vi "Write Setpoint.vi"(8 "error in (no error)":errorcluster, 10 "ILC in":refnum<class "ILC.lvclass">, 11 "ILC Actuator Cylinder in":refnum<class "ILC Actuator Cylinder.lvclass">) -> (0 "error out":errorcluster, 1 "Cylinder Results":T1, 2 "ILC out":refnum<class "ILC.lvclass">, 3 "ILC Actuator Cylinder out":refnum<class "ILC Actuator Cylinder.lvclass">)   [LabVIEW 2015, in "ILC Actuator Cylinder.lvclass"]
uses:
  ILC Actuator Cylinder.lvclass
  <userlib>/Common/ILC/ILC/ILC.lvclass
  Typedefs/Cylinder Results.ctl
  ILC Actuator Cylinder.lvclass/ILC Actuator Cylinder.ctl
  ILC DAC/ILC DAC/ILC DAC.lvclass
  Calculators/Force To Pressure Servo Valve Voltage/Force To Pressure Servo Valve Voltage.lvclass
  Typedefs/FAMT Typedefs.lvlib
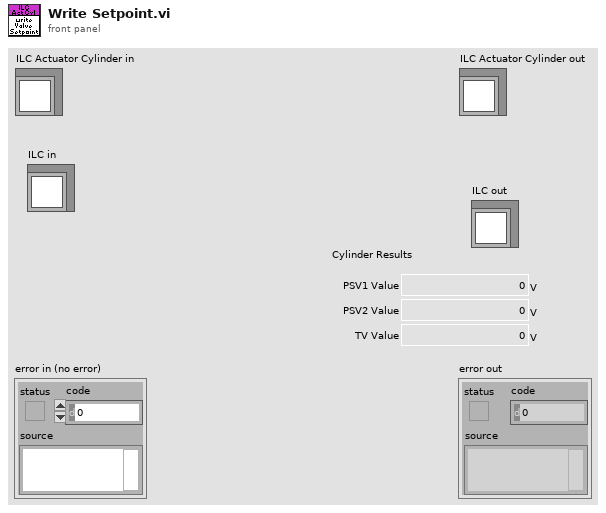
[diagram p1: front panel]
types:
  T1 = typedef "FAMT Typedefs.lvlib/Cylinder Results.ctl" = cluster{"PSV1 Value":dbl[unit], "PSV2 Value":dbl[unit], "TV Value":dbl[unit]}
  T2 = typedef "FAMT Typedefs.lvlib/Pressure Servo Valve Settings.ctl" = cluster{"Center Point":dbl[unit], "Area":dbl, "PA to PSI":dbl, "Off Value":dbl}
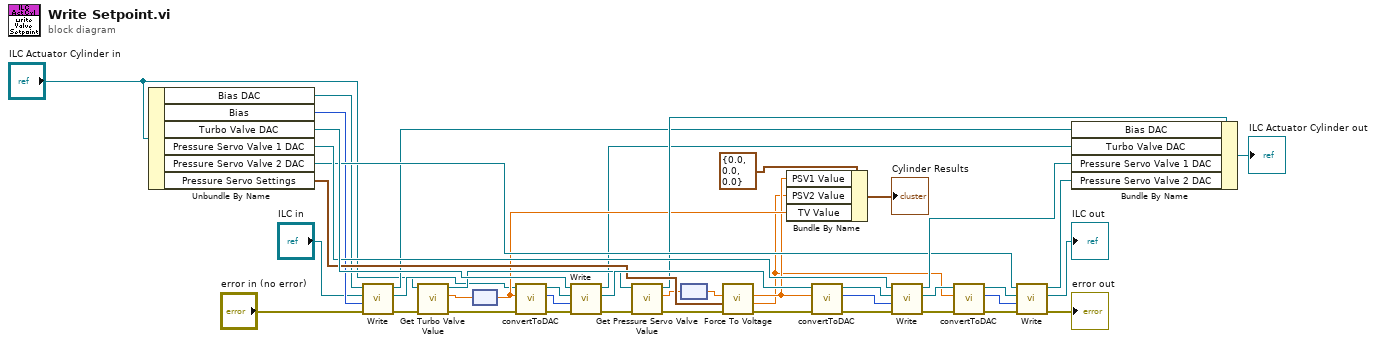
[diagram p0: block diagram]
diagram:
  n1 = Unbundle By Name("ILC Actuator Cylinder in") -> ("Bias DAC"=w9:refnum<class "ILC DAC.lvclass">, "Bias"=w6:u16, "Turbo Valve DAC"=w40:refnum<class "ILC DAC.lvclass">, "Pressure Servo Valve 1 DAC"=w37:refnum<class "ILC DAC.lvclass">, "Pressure Servo Valve 2 DAC"=w31:refnum<class "ILC DAC.lvclass">, "Pressure Servo Settings"=w24:T2)
  n2 = call-dynamic "Write.vi"("error in (no error)"="error in (no error)", "Value"=w6, "ILC in"="ILC in", "ILC DAC in"=w9) -> ("error out"=w2:errorcluster, "ILC out"=w4:refnum<class "ILC.lvclass">, "ILC DAC out"=w8:refnum<class "ILC DAC.lvclass">)  [unwired: 5 in]
  n3 = call-dynamic "Get Turbo Valve Value.vi"("error in (no error)"=w2, "ILC Actuator Cylinder in"="ILC Actuator Cylinder in") -> ("error out"=w23:errorcluster, "Value"=w22:dbl, "ILC Actuator Cylinder out"=w19:refnum<class "ILC Actuator Cylinder.lvclass">)  [unwired: 7 in]
  n4 = node(w22) -> (w12:dbl[unit])
  n5 = call <userlib>:"convertToDAC.vi"("error in (no error)"=w23, "Voltage"=w12, "ILC in"=w4) -> ("error out"=w30:errorcluster, "Counts"=w41:u16, "ILC out"=w42:refnum<class "ILC.lvclass">)  [unwired: 6 in]
  n6 = call-dynamic "Write.vi"("error in (no error)"=w30, "Value"=w41, "ILC in"=w42, "ILC DAC in"=w40) -> ("error out"=w20:errorcluster, "ILC out"=w39:refnum<class "ILC.lvclass">, "ILC DAC out"=w1:refnum<class "ILC DAC.lvclass">)  [unwired: 5 in]
  n7 = call-dynamic "Get Pressure Servo Valve Value.vi"("error in (no error)"=w20, "ILC Actuator Cylinder in"=w19) -> ("error out"=w21:errorcluster, "Value"=w15:dbl, "ILC Actuator Cylinder out"=w18:refnum<class "ILC Actuator Cylinder.lvclass">)  [unwired: 7 in]
  n8 = node(w15) -> (w16:dbl[unit])
  n9 = call "Force To Voltage.vi"("error in (no error)"=w21, "Pressure Servo Settings"=w24, "Force"=w16) -> ("error out"=w25:errorcluster, "Voltage 2"=w10:dbl[unit], "Voltage 1"=w11:dbl[unit])  [unwired: 5 in, 1 out]
  n10 = Bundle By Name(cluster=T1 {"PSV1 Value"=0.0, "PSV2 Value"=0.0, "TV Value"=0.0} ("Cylinder Results"), "PSV1 Value"=w11, "PSV2 Value"=w10, "TV Value"=w12) -> (→"Cylinder Results":T1)
  n11 = call <userlib>:"convertToDAC.vi"("error in (no error)"=w25, "Voltage"=w11, "ILC in"=w39) -> ("error out"=w29:errorcluster, "Counts"=w17:u16, "ILC out"=w38:refnum<class "ILC.lvclass">)  [unwired: 6 in]
  n12 = call-dynamic "Write.vi"("error in (no error)"=w29, "Value"=w17, "ILC in"=w38, "ILC DAC in"=w37) -> ("error out"=w28:errorcluster, "ILC out"=w35:refnum<class "ILC.lvclass">, "ILC DAC out"=w36:refnum<class "ILC DAC.lvclass">)  [unwired: 5 in]
  n13 = call <userlib>:"convertToDAC.vi"("error in (no error)"=w28, "Voltage"=w10, "ILC in"=w35) -> ("error out"=w27:errorcluster, "Counts"=w33:u16, "ILC out"=w34:refnum<class "ILC.lvclass">)  [unwired: 6 in]
  n14 = call-dynamic "Write.vi"("error in (no error)"=w27, "Value"=w33, "ILC in"=w34, "ILC DAC in"=w31) -> ("error out"=→"error out":errorcluster, "ILC out"=→"ILC out":refnum<class "ILC.lvclass">, "ILC DAC out"=w32:refnum<class "ILC DAC.lvclass">)  [unwired: 5 in]
  n15 = Bundle By Name(cluster=w18, "Bias DAC"=w8, "Turbo Valve DAC"=w1, "Pressure Servo Valve 1 DAC"=w36, "Pressure Servo Valve 2 DAC"=w32) -> (→"ILC Actuator Cylinder out":refnum<class "ILC Actuator Cylinder.lvclass">)
